vi "S2C_OM8257_Proc_Initialize.vi"(7 "Local?":bool, 8 "Error In":errorcluster, 10 "Command":string, 11 "JSON String":string) -> (0 "Error Out":errorcluster, 2 "Response":variant)   [LabVIEW 2015]
uses:
  S2C_OM8257_Proc_Globals.vi
  <instrlib>/Associated Research 82XX/Associated Research 82XX.lvlib
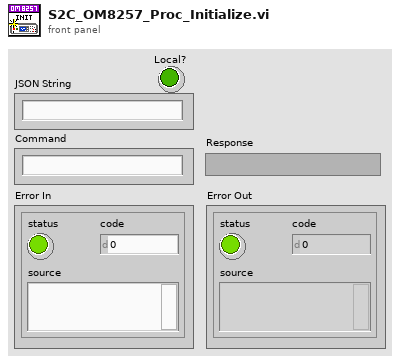
[diagram p1: front panel]
types:
  T1 = cluster{"Baud Rate (9600)":u32, "Parity (None)":u16, "Data Bits (8)":u16, "Stop Bits (1)":u16, "Flow Control (None)":u16}
  T2 = cluster{"Resource Name":string, "Baud Rate":u32, "Data Bits":u16, "Parity":u16, "Stop Bits":u16, "Flow Control":u16, "Timeout":u32, "Reset":bool}
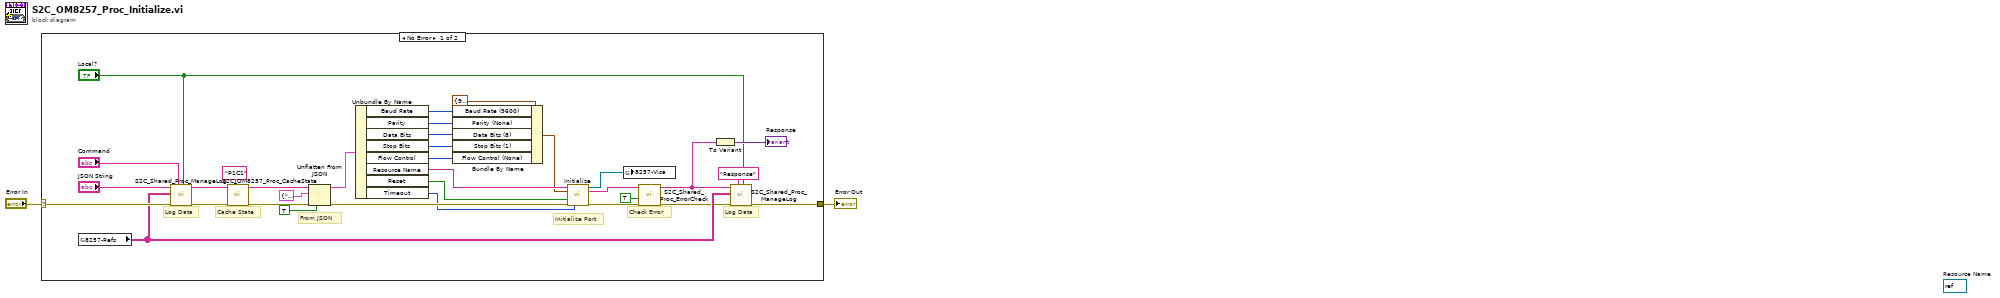
[diagram p0: block diagram]
diagram:
  (unwired) refnum<visa-resource-name> refnum  # Resource Name
  n1 = case shown="No Error" "Error In" {
    selector: "Error In" -> [w31 w36]
    tunnel: [w29 w36] -> w1
    frame No Error {
      # "Check Error"
      # "Initialize Port"
      # "Cache State"
      # "Log Data"
      # "Log Data"
      # "From JSON"
      n2 = global read "S2C_OM8257_Proc_Globals.vi" "8257-Refs"() -> (w21:string[][])
      n3 = call "S2C_Shared_Proc_ManageLog.vi"("Local?"="Local?", "Command"="Command", "Error In"=w31, "Refs"=w21, "Data In"="JSON String") -> ("Error Out"=w27:errorcluster, "Data Out"=w26:string)  [unwired: 5 in]
      n4 = call "S2C_OM8257_Proc_CacheState.vi"("Label"="P1C1", "Error In"=w27, "Data In"=w26) -> ("Error Out"=w24:errorcluster, "Data Out"=w25:string)  [unwired: 7 in]
      n5 = Unflatten From JSON(JSON string=w25, type and defaults=T2 {"Resource Name"="", "Baud Rate"=0, "Data Bits"=0, "Parity"=0, "Stop Bits"=10, "Flow Control"=0, "Timeout"=0, "Reset"=FALSE} ("P1C1"), default null elements? (F)=TRUE, error in (no error)=w24) -> (value=w34:T2, error out=w32:errorcluster)  [unwired: 3 in]
      n6 = Unbundle By Name(w34) -> ("Baud Rate"=w18:u32, "Parity"=w17:u16, "Data Bits"=w16:u16, "Stop Bits"=w15:u16, "Flow Control"=w14:u16, "Resource Name"=w11:string, "Reset"=w12:bool, "Timeout"=w13:u32)
      n7 = Bundle By Name(cluster=T1 {"Baud Rate (9600)"=9600, "Parity (None)"=0, "Data Bits (8)"=8, "Stop Bits (1)"=10, "Flow Control (None)"=0} ("Serial Configuration"), "Baud Rate (9600)"=w18, "Parity (None)"=w17, "Data Bits (8)"=w16, "Stop Bits (1)"=w15, "Flow Control (None)"=w14) -> (w10:T1)
      n8 = call <instrlib>:"Initialize.vi"("VISA resource name"=w11, "Serial Configuration"=w10, "Reset (True)"=w12, "error in (no error)"=w32, "Timeout (10000 ms)"=w13) -> ("VISA resource name out"=w3:refnum<visa-resource-name>, "Firmware Version"=w8:string, "error out"=w9:errorcluster)  [unwired: 8 in]
      n9 = global write "S2C_OM8257_Proc_Globals.vi" "8257-Visa"(w3) -> ()
      n10 = call "S2C_Shared_Proc_ErrorCheck.vi"("Error In"=w9, "ExpReply?"=TRUE, "Reply Text"=w8) -> ("Error Out"=w6:errorcluster, "Status"=w4:string)  [unwired: 7 in]
      n11 = To Variant(anything=w4) -> (Variant=→"Response":variant)
      n12 = call "S2C_Shared_Proc_ManageLog.vi"("Local?"="Local?", "Command"="Response", "Error In"=w6, "Refs"=w21, "Data In"=w4) -> ("Error Out"=w29:errorcluster)  [unwired: 5 in, 1 out]
    }
    frame Error {
    }
  }
  "Error Out" <- w1
